vi "MM9.i attribute.vi"(0 "VI Refnum":refnum<vi>, 2 "CLASS.i attribute":T1={"UsedObjs"=[], "ActScanStep"=[], "AbortRequest"=FALSE, "StopRequest"=FALSE, "# cycles"=0, "Connected"=FALSE, "MMStatus"=enum."config", "# data"=0, "DIMServices"={"MM6StatusString"="", "MM6StatusID"=-1, "discArchiver"="", "discArchiverID"=-1, "eventBuilder"="", "eventBuilderID"=-1, "GUIIDString"="", "GUIIDStringID"=-1}, "dataFile"="", "PGRunning"=0, "ConfigData"={"GenConfig"={"Mode"=0, "Logs"=[]}, "Configs"=[]}, "ExtraDataSets"=[]} {"ConfigData"."Configs"."CleanDev"."CleanData"."Time" format="%.3f"; "ConfigData"."Configs"."CleanDev"."CleanData"."Minus" format="%.2f"; "ConfigData"."Configs"."CleanDev"."CleanData"."Plus" format="%.2f"; "ConfigData"."Configs"."CleanDev"."CleanData"."Center" format="%.4f"; "ConfigData"."Configs"."CleanDev"."CleanData"."Amp" format="%.2f"; "ConfigData"."Configs"."Delays"."Delay" format="%.2f"; "ConfigData"."Configs"."Specials"."Data" format="%.2f"; "ConfigData"."Configs"."FreqDevs"."Time" format="%.3f"; "ConfigData"."Configs"."FreqDevs"."CenterFreq" format="%.4f"; "ConfigData"."Configs"."FreqDevs"."Amp" format="%.2f"; "ConfigData"."Configs"."Scans"."Values" format="%.2f"}, 3 "Action":T20(ring), 5 "error in (no error)":errorcluster) -> (14 "VI Refnum out":refnum<vi>, 16 "CLASS.i attribute out":T1={"UsedObjs"=[], "ActScanStep"=[], "AbortRequest"=FALSE, "StopRequest"=FALSE, "# cycles"=0, "Connected"=FALSE, "MMStatus"=enum."config", "# data"=0, "DIMServices"={"MM6StatusString"="", "MM6StatusID"=-1, "discArchiver"="", "discArchiverID"=-1, "eventBuilder"="", "eventBuilderID"=-1, "GUIIDString"="", "GUIIDStringID"=-1}, "dataFile"="", "PGRunning"=0, "ConfigData"={"GenConfig"={"Mode"=0, "Logs"=[]}, "Configs"=[]}, "ExtraDataSets"=[]} {"ConfigData"."Configs"."CleanDev"."CleanData"."Time" format="%.3f"; "ConfigData"."Configs"."CleanDev"."CleanData"."Minus" format="%.2f"; "ConfigData"."Configs"."CleanDev"."CleanData"."Plus" format="%.2f"; "ConfigData"."Configs"."CleanDev"."CleanData"."Center" format="%.4f"; "ConfigData"."Configs"."CleanDev"."CleanData"."Amp" format="%.2f"; "ConfigData"."Configs"."Delays"."Delay" format="%.2f"; "ConfigData"."Configs"."Specials"."Data" format="%.2f"; "ConfigData"."Configs"."FreqDevs"."Time" format="%.3f"; "ConfigData"."Configs"."FreqDevs"."CenterFreq" format="%.4f"; "ConfigData"."Configs"."FreqDevs"."Amp" format="%.2f"; "ConfigData"."Configs"."Scans"."Values" format="%.2f"}, 19 "error out":errorcluster)   [LabVIEW 2014, in "MM9.lvlib"]
doc: "This is a so-called functional global variable. It manages the access to a global variable in a thread-safe way. \n\nHere the attribute data of all instances of THIS class are stored. This is done for performance reasons.\n\nLicense Agreement for this software:\n\nCopyright (C)\nGesellschaft für Schwerionenforschung, GSI\nPlanckstr. 1\n64291 Darmstadt\nGermany\n\nContact: D.Beck@gsi.de \n\nThis program is free software; you can redistribute it and/or modify it under the terms of the GNU General Public License as published by the Free Software Foundation; either version 2 of the license, or (at your option) any later version.\n\nThis program is distributed in the hope that it will be useful, but WITHOUT ANY WARRANTY; without even the implied warranty of MERCHANTABILITY or FITNESS FOR A PARTICULAR PURPOSE. See the GNU General License for more details (http://www.gnu.org).\n\nGesellschaft für Schwerionenforschung, GSI\nPlanckstr. 1, 64291 Darmstadt, Germany\nFor all questions and ideas contact: M.Richter@gsi.de, H.Brand@gsi.de or D.Beck@gsi.de.\nLast update: 17-JUN-2004"
uses:
  MM9.lvlib
  MM9.i attribute.ctl
  MM9.status.ctl
  CS_DigitalIO/PPG_ABC/PPG_ABC.PG_Running.ctl
  LEBITDefs9/LEBITDefs.ConfigData.ctl
  LEBITDefs9/LEBITDefs.GenConfig.ctl
  LEBITDefs9/LEBITDefs.Log.ctl
  LEBITDefs9/LEBITDefs.OneConfig.ctl
  LEBITDefs9/LEBITDefs.MCA.ctl
  LEBITDefs9/LEBITDefs.Timing.ctl
  LEBITDefs9/LEBITDefs.Timetable.ctl
  LEBITDefs9/LEBITDefs.Memory.ctl
  LEBITDefs9/LEBITDefs.ScanDev.ctl
  LEBITDefs9/LEBITDefs.FreqDev.ctl
  LEBITDefs9/LEBITDefs.CleanDev.ctl
  LEBITDefs9/LEBITDefs.CleanDataType.ctl
  LEBITDefs9/LEBITDefs.Special.ctl
  LEBITDefs9/LEBITDefs.Delay.ctl
  LEBITDefs9/LEBITDefs.DAC.ctl
  LEBITDefs9/LEBITDefs.ExtraData.ctl
  CS_Core/CSSystem/CoreDefs/CoreDefs.error_type.ctl
  CS_Core/CSSystem/CoreLib/CoreLib.lvlib
  CS_DigitalIO/PPG_ABC/PPG_ABC.lvlib
  LEBITDefs9/LEBITDefs9.lvlib
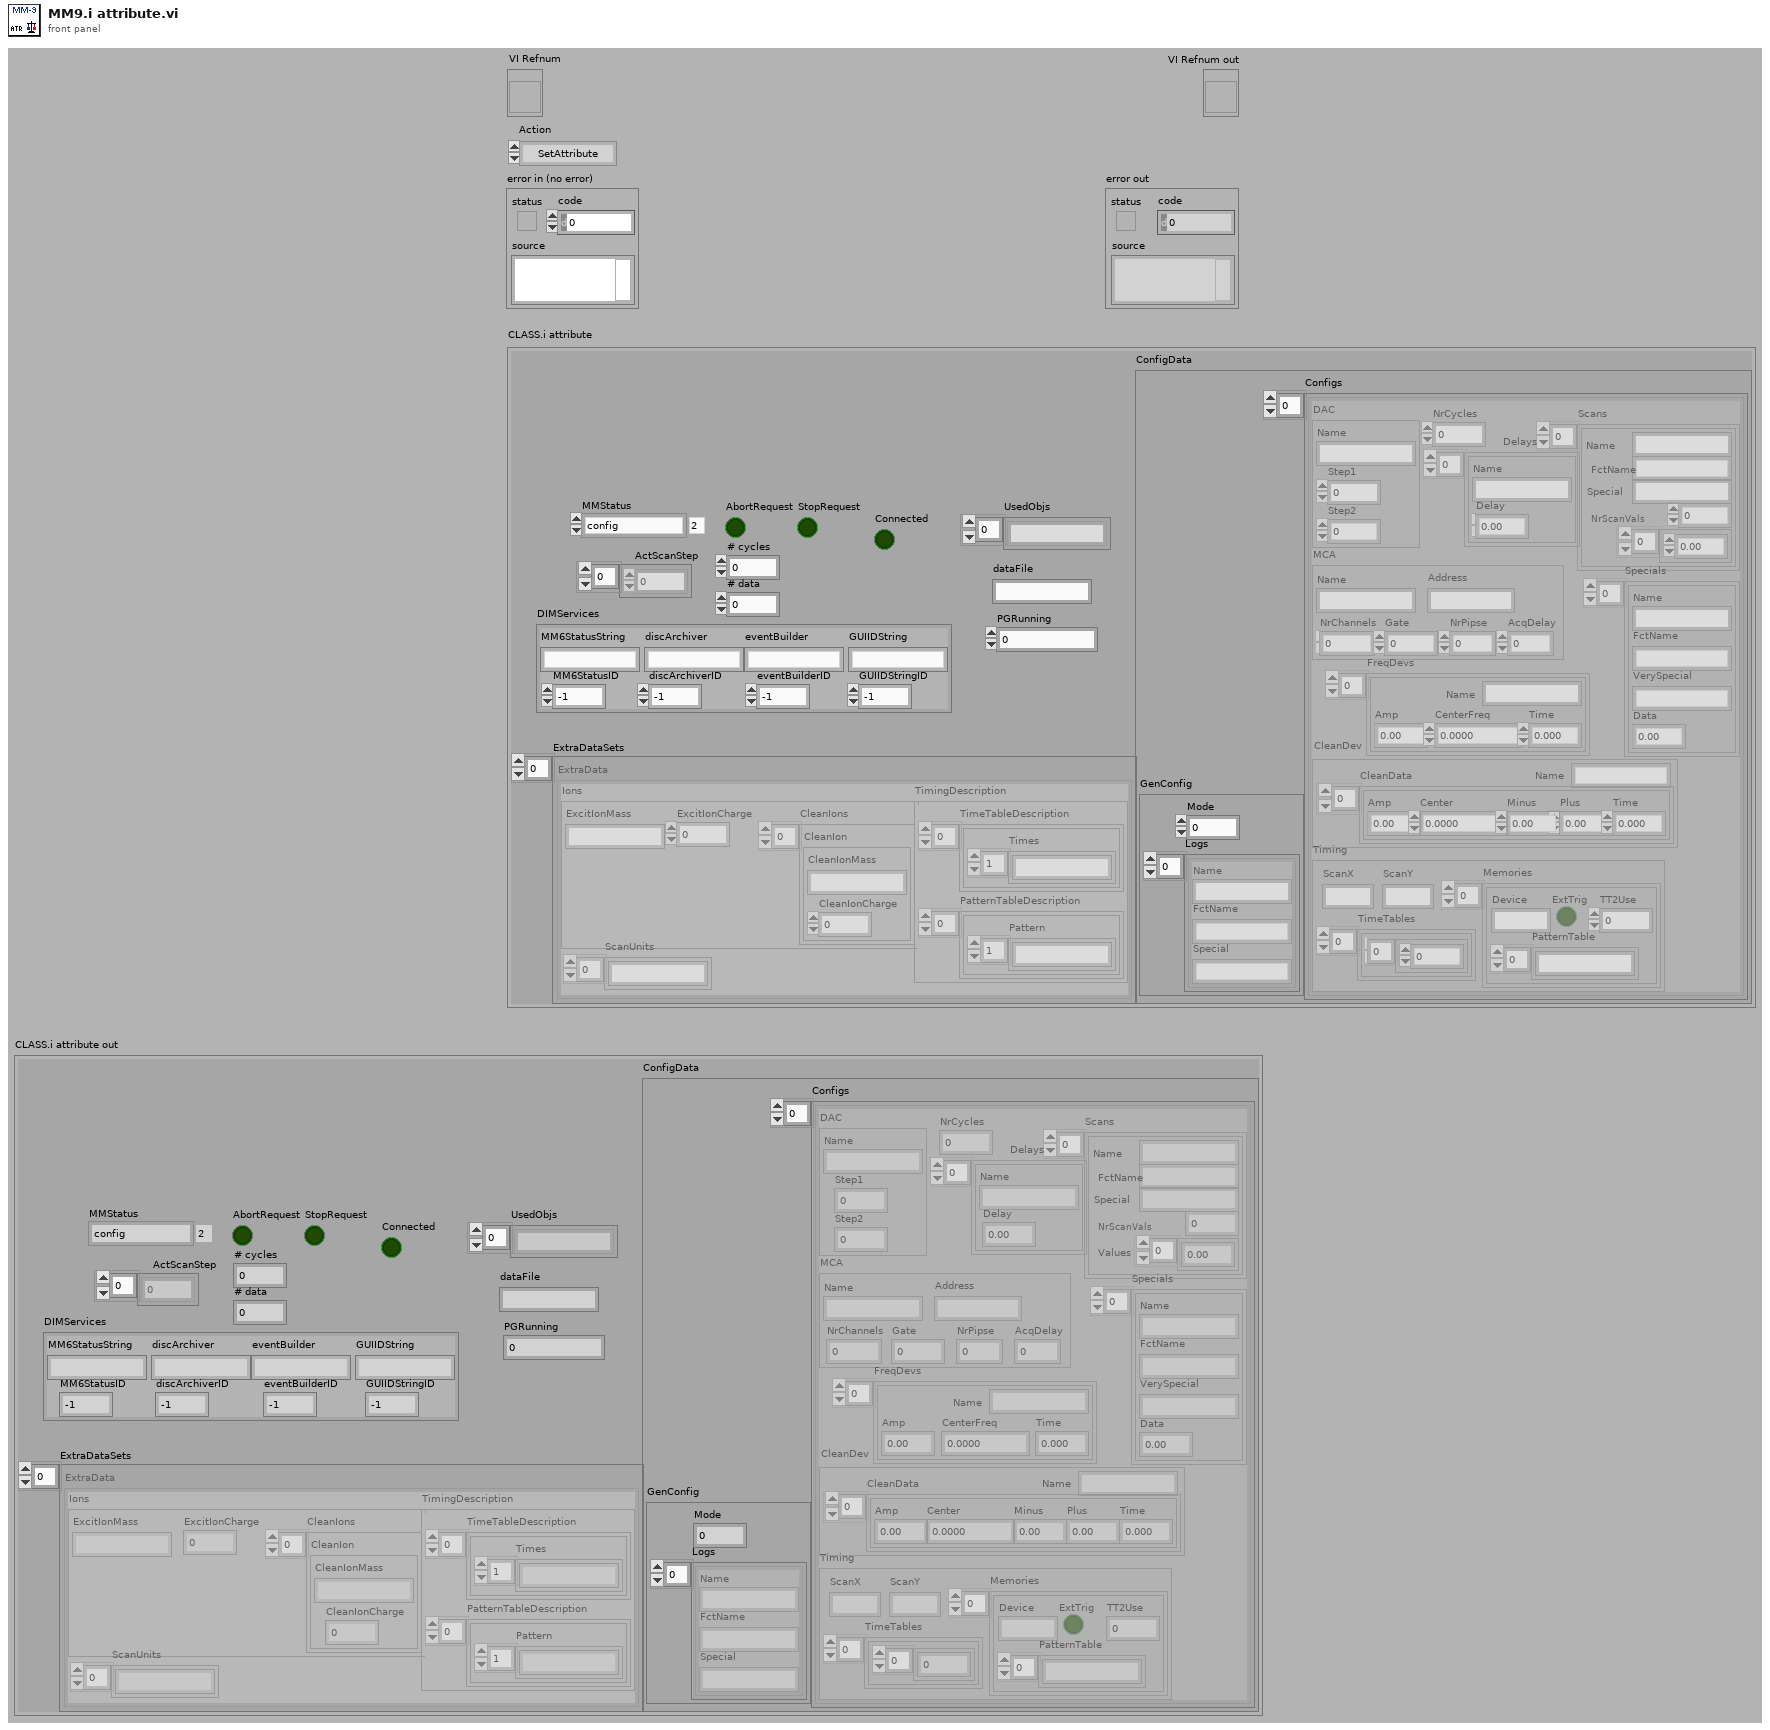
[diagram p1: front panel]
types:
  T1 = typedef "MM9.lvlib/MM9.i attribute.ctl" = cluster{"UsedObjs":string[], "ActScanStep":i32[], "AbortRequest":bool, "StopRequest":bool, "# cycles":i32, "Connected":bool, "MMStatus":T2, "# data":i32, "DIMServices":cluster{"MM6StatusString":string, "MM6StatusID":i32, "discArchiver":string, "discArchiverID":i32, "eventBuilder":string, "eventBuilderID":i32, "GUIIDString":string, "GUIIDStringID":i32}, "dataFile":string, "PGRunning":T3, "ConfigData":T4, "ExtraDataSets":T19}
  T2 = typedef "MM9.lvlib/MM9.status.ctl" = enum16{"loaded", "load_error", "config", "config_error", "init", "init_error", "data_reset", "data_reset_error", "running", "start_error", "run_error", "abort_requested", "aborted", "stop_requested", "stopped", "stop_error", "Connected", "NOTConnected"}
  T3 = typedef "PPG_ABC.lvlib/PPG_ABC.PG_Running.ctl" = i32
  T4 = typedef "LEBITDefs9.lvlib/LEBITDefs.ConfigData.ctl" = cluster{"GenConfig":T5, "Configs":T7[]}
  T5 = typedef "LEBITDefs9.lvlib/LEBITDefs.GenConfig.ctl" = cluster{"Mode":i32, "Logs":T6[]}
  T6 = typedef "LEBITDefs9.lvlib/LEBITDefs.Log.ctl" = cluster{"Name":string, "FctName":string, "Special":string}
  T7 = typedef "LEBITDefs9.lvlib/LEBITDefs.OneConfig.ctl" = cluster{"MCA":T8, "Timing":T9, "Scans":T12[], "FreqDevs":T13[], "CleanDev":T14, "NrCycles":i32, "Specials":T16[], "Delays":T17[], "DAC":T18}
  T8 = typedef "LEBITDefs9.lvlib/LEBITDefs.MCA.ctl" = cluster{"Name":string, "Address":string, "NrChannels":i32, "Gate":i32, "NrPipse":i32, "AcqDelay":i32}
  T9 = typedef "LEBITDefs9.lvlib/LEBITDefs.Timing.ctl" = cluster{"TimeTables":cluster{"TimeTable":T10}[], "Memories":T11[], "ScanX":string, "ScanY":string}
  T10 = typedef "LEBITDefs9.lvlib/LEBITDefs.Timetable.ctl" = dbl[]
  T11 = typedef "LEBITDefs9.lvlib/LEBITDefs.Memory.ctl" = cluster{"Device":string, "ExtTrig":bool, "TT2Use":i32, "PatternTable":string[]}
  T12 = typedef "LEBITDefs9.lvlib/LEBITDefs.ScanDev.ctl" = cluster{"Name":string, "FctName":string, "Values":dbl[], "NrScanVals":i32, "Special":string}
  T13 = typedef "LEBITDefs9.lvlib/LEBITDefs.FreqDev.ctl" = cluster{"Name":string, "Amp":dbl, "CenterFreq":dbl, "Time":dbl}
  T14 = typedef "LEBITDefs9.lvlib/LEBITDefs.CleanDev.ctl" = cluster{"Name":string, "CleanData":T15[]}
  T15 = typedef "LEBITDefs9.lvlib/LEBITDefs.CleanDataType.ctl" = cluster{"Amp":dbl, "Center":dbl, "Plus":dbl, "Minus":dbl, "Time":dbl}
  T16 = typedef "LEBITDefs9.lvlib/LEBITDefs.Special.ctl" = cluster{"Name":string, "FctName":string, "VerySpecial":string, "Data":dbl}
  T17 = typedef "LEBITDefs9.lvlib/LEBITDefs.Delay.ctl" = cluster{"Name":string, "Delay":dbl}
  T18 = typedef "LEBITDefs9.lvlib/LEBITDefs.DAC.ctl" = cluster{"Name":string, "Step1":i32, "Step2":i32}
  T19 = typedef "LEBITDefs9.lvlib/LEBITDefs.ExtraData.ctl" = cluster{"Ions":cluster{"ExcitIonMass":string, "ExcitIonCharge":i32, "CleanIons":cluster{"CleanIonMass":string, "CleanIonCharge":i32}[]}, "TimingDescription":cluster{"TimeTableDescription":cluster{"Times":string[]}[], "PatternTableDescription":cluster{"Pattern":string[]}[]}, "ScanUnits":string[]}[]
  T20 = enum16{"SetAttribute", "GetAttribute", "CreateAttribute", "DestroyAttribute", "DestroyAllAtributes"}
  T21 = typedef "CoreDefs.error_type.ctl" = enum16{"no error", "can't load process", "can't unload process", "process does not exist", "can't install process", "can't remove process", "unknown function", "time out", "can't execute function", "duplicate queue name", "super not found", "caller queue invalid", "can't ping process", "unknown error", "VISA Error", "VISA timeout", "GPIB timeout", "GPIB error", "communication error", "data type mismatch", "can't read data from OPC server", "can't write data to OPC server", "OET error", "function not implemented", "process already exists", "invalid Shared Variable name", "error writing Shared Variable", "error reading Shared Variable", "invalid client name", "corrupt database", "unknown class", "call not authorized", "parameter out of range", "OET timeout: can't get data to modify", "invalid queue name", "requested operation incompatible with current state", "event undefined", "event disabled", "state undefined", "caller is not a friend", "EventBuilder: bad eventID", "EventBuilder: no DAQ devices", "a thread must not stop itself", "UNUSED ELEMENT4", "DiscArchiver: eventData incomplete", "DiscArchiver: eventData does not belong to run", "DiscArchiver: can't open file", "DiscArchiver: can't write to file", "DiscArchiver: available disc space low", "can't acquire semaphore", "error reading data from database", "notifier object is not existing", "can't register process", "can't unregister process", "illegal event type", "object disabled", "object already exists", "can't change state", "Instrument not found", "no connection to remote node", "invalid reference", "N/A", "UNUSED ELEMENT 1", "element not found", "illegal TCP/IP connection detected", "object does not exist", "invalid access ID", "unknown CS system", "invalid privilige", "unsupported data type", "unsupported server type", "IO server already exists", "Shared Variable already exists"}
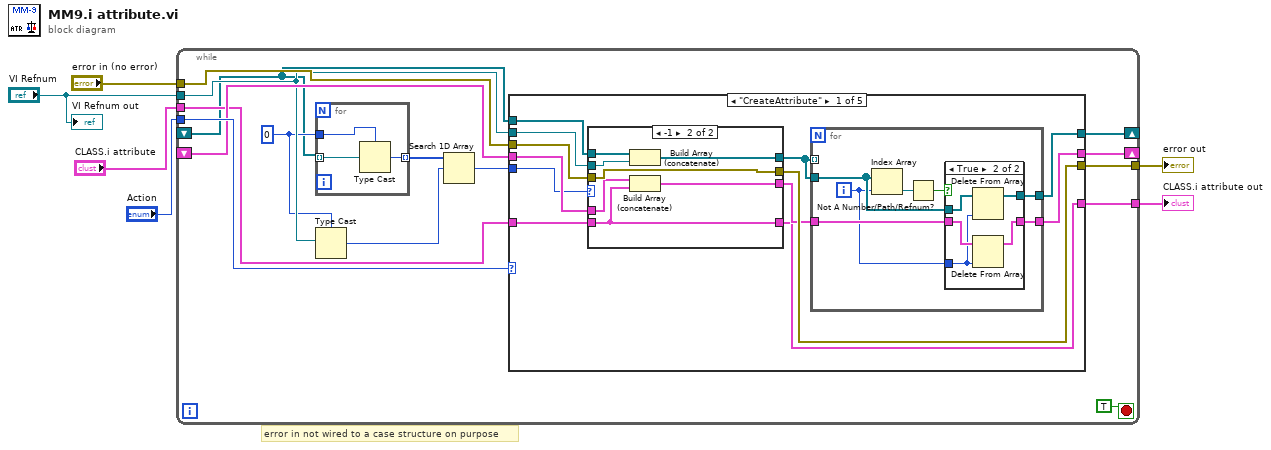
[diagram p0: block diagram]
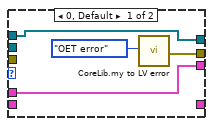
[diagram p3: hidden frame]
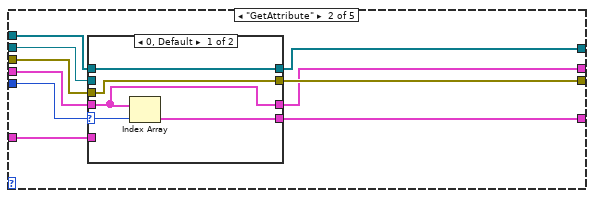
[diagram p4: hidden frame]
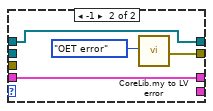
[diagram p5: hidden frame]
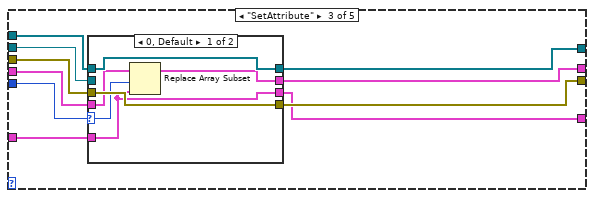
[diagram p6: hidden frame]
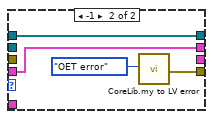
[diagram p7: hidden frame]
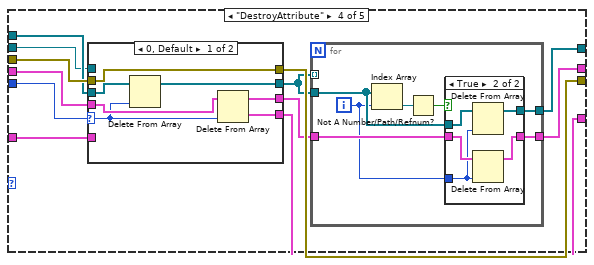
[diagram p8: hidden frame]
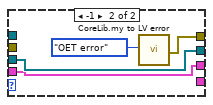
[diagram p10: hidden frame]
diagram:
  # "error in not wired to a case structure on purpose"
  n1 = while {
    shift-right: [w15] -> _
    shift-left: _ -> [w16]
    tunnel: "Action" -> [w20]
    shift-right: [w17] -> _
    shift-left: _ -> [w7]
    tunnel: "error in (no error)" -> [w19]
    tunnel: [w18] -> w4
    tunnel: "CLASS.i attribute" -> [w14]
    tunnel: [w12] -> w2
    tunnel: "VI Refnum" -> [w10]
    stop <- TRUE stop-if-true
    w9 = 0
    n2 = for {
      tunnel: w9 -> [w24]
      tunnel: [w23] -> w8 mode=indexing
      tunnel: w7 -> [w22] mode=indexing
      n3 = Type Cast(type=w24, x=w22) -> (*(type *) &x=w23:i32)
    }
    n4 = Type Cast(type=w9, x=w10) -> (*(type *) &x=w11:i32)
    n5 = Search 1D Array(1D array=w8, element=w11) -> (index of element=w13:i32)  [unwired: 1 in]
    n6 = case shown="\"CreateAttribute\"" w20 {
      tunnel: w7 -> [w34 w69 w88 w110 _]
      tunnel: w10 -> [w33 w67 w86 w109 _]
      tunnel: w19 -> [w36 w71 w90 w112 w138]
      tunnel: [w35 w70 w89 w111 w138] -> w18
      tunnel: [w29 w68 w87 w104 _] -> w17
      tunnel: w16 -> [w32 w66 w85 w108 _]
      tunnel: [w27 w65 w84 w103 _] -> w15
      tunnel: w14 -> [w31 w64 w83 w107 _]
      tunnel: w13 -> [w30 w63 w82 w106 _]
      tunnel: [w25 w62 w81 w101 _] -> w12
      frame "CreateAttribute" {
        n7 = case shown="-1" w30 {
          tunnel: w36 -> [_ w61]
          tunnel: [w53 w61] -> w35
          tunnel: w34 -> [w52 w60]
          tunnel: [w52 w59] -> w26
          tunnel: w33 -> [_ w58]
          tunnel: w32 -> [w51 w57]
          tunnel: [w51 w56] -> w28
          tunnel: w31 -> [_ w55]
          tunnel: [_ w55] -> w25
          frame 0, Default {
            n8 = call "CoreLib.my to LV error.vi"("ErrorTypes"=CoreDefs.error_type."OET error") -> ("myErrorCluster"=w53:errorcluster)  [unwired: 17 in, 1 out]
          }
          frame -1 {
            n9 = Build Array (concatenate)(w60, w58) -> (w59:refnum<vi>[])
            n10 = Build Array (concatenate)(w57, w55) -> (w56:T1[])
          }
        }
        n11 = for {
          tunnel: w26 -> [w39]
          tunnel: [w38] -> w29
          tunnel: [w43] -> w27
          tunnel: w28 -> [w42]
          tunnel: w26 -> [_] mode=indexing
          i -> [w37]
          n12 = Index Array(array=w39, index=w37) -> (element=w40:refnum<vi>)
          n13 = Not A Number/Path/Refnum?(number/path/refnum=w40) -> (NaN/Path/Refnum?=w41:bool)
          n14 = case shown="True" w41 {
            tunnel: [w45 w50] -> w43
            tunnel: w42 -> [w45 w49]
            tunnel: [w44 w47] -> w38
            tunnel: w39 -> [w44 w48]
            tunnel: w37 -> [_ w46]
            frame False {
            }
            frame True {
              n15 = Delete From Array(array=w48, index=w46) -> (array with subset deleted=w47:refnum<vi>[])  [unwired: 1 in, 1 out]
              n16 = Delete From Array(array=w49, index=w46) -> (array with subset deleted=w50:T1[])  [unwired: 1 in, 1 out]
            }
          }
        }
      }
      frame "GetAttribute" {
        n17 = case shown="0, Default" w63 {
          selector: w63 -> [w74 _]
          tunnel: w71 -> [w76 _]
          tunnel: [w76 w79] -> w70
          tunnel: w69 -> [w75 w78]
          tunnel: [w75 w78] -> w68
          tunnel: w67 -> [_ _]
          tunnel: w66 -> [w73 w77]
          tunnel: [w73 w77] -> w65
          tunnel: w64 -> [_ _]
          tunnel: [w72 _] -> w62
          frame 0, Default {
            n18 = Index Array(array=w73, index=w74) -> (element=w72:T1)
          }
          frame -1 {
            n19 = call "CoreLib.my to LV error.vi"("ErrorTypes"=CoreDefs.error_type."OET error") -> ("myErrorCluster"=w79:errorcluster)  [unwired: 17 in, 1 out]
          }
        }
      }
      frame "SetAttribute" {
        n20 = case shown="0, Default" w82 {
          selector: w82 -> [w92 _]
          tunnel: w90 -> [w96 _]
          tunnel: [w96 w99] -> w89
          tunnel: w88 -> [w95 w98]
          tunnel: [w95 w98] -> w87
          tunnel: w86 -> [_ _]
          tunnel: w85 -> [w94 w97]
          tunnel: [w93 w97] -> w84
          tunnel: w83 -> [w91 _]
          tunnel: [w91 _] -> w81
          frame 0, Default {
            n21 = Replace Array Subset(array=w94, new element=w91, index=w92) -> (w93:T1[])
          }
          frame -1 {
            n22 = call "CoreLib.my to LV error.vi"("ErrorTypes"=CoreDefs.error_type."OET error") -> ("myErrorCluster"=w99:errorcluster)  [unwired: 17 in, 1 out]
          }
        }
      }
      frame "DestroyAttribute" {
        n23 = case shown="0, Default" w106 {
          selector: w106 -> [w129 _]
          tunnel: w112 -> [w133 _]
          tunnel: [w133 w136] -> w111
          tunnel: w110 -> [w132 w135]
          tunnel: [w131 w135] -> w102
          tunnel: w109 -> [_ _]
          tunnel: w108 -> [w130 w134]
          tunnel: [w128 w134] -> w105
          tunnel: w107 -> [_ _]
          tunnel: [w127 _] -> w101
          frame 0, Default {
            n24 = Delete From Array(array=w132, index=w129) -> (array with subset deleted=w131:refnum<vi>[])  [unwired: 1 in, 1 out]
            n25 = Delete From Array(array=w130, index=w129) -> (deleted portion=w127:T1, array with subset deleted=w128:T1[])  [unwired: 1 in]
          }
          frame -1 {
            n26 = call "CoreLib.my to LV error.vi"("ErrorTypes"=CoreDefs.error_type."OET error") -> ("myErrorCluster"=w136:errorcluster)  [unwired: 17 in, 1 out]
          }
        }
        n27 = for {
          tunnel: w102 -> [w115]
          tunnel: [w114] -> w104
          tunnel: [w119] -> w103
          tunnel: w105 -> [w118]
          tunnel: w102 -> [_] mode=indexing
          i -> [w113]
          n28 = Index Array(array=w115, index=w113) -> (element=w116:refnum<vi>)
          n29 = Not A Number/Path/Refnum?(number/path/refnum=w116) -> (NaN/Path/Refnum?=w117:bool)
          n30 = case shown="True" w117 {
            tunnel: [w121 w126] -> w119
            tunnel: w118 -> [w121 w125]
            tunnel: [w120 w123] -> w114
            tunnel: w115 -> [w120 w124]
            tunnel: w113 -> [_ w122]
            frame False {
            }
            frame True {
              n31 = Delete From Array(array=w124, index=w122) -> (array with subset deleted=w123:refnum<vi>[])  [unwired: 1 in, 1 out]
              n32 = Delete From Array(array=w125, index=w122) -> (array with subset deleted=w126:T1[])  [unwired: 1 in, 1 out]
            }
          }
        }
      }
      frame "DestroyAllAtributes" {
      }
    }
  }
  "error out" <- w4
  "CLASS.i attribute out" <- w2
  "VI Refnum out" <- "VI Refnum"
